vi "ReversedEngineering EvaluateStateActions.vi"(1 "SubViNames":string[](array[string]), 2 "StateDiagramSerachActions":T2, 5 "error in":errorcluster) -> (15 "StateActions":string[](array[string]), 19 "error out":errorcluster)   [LabVIEW 2016]
uses:
  <resource>/Framework/Providers/Open_GDS/UML/ReversedEngineering/ReversedEngineering StateAnalyseVIAction.ctl
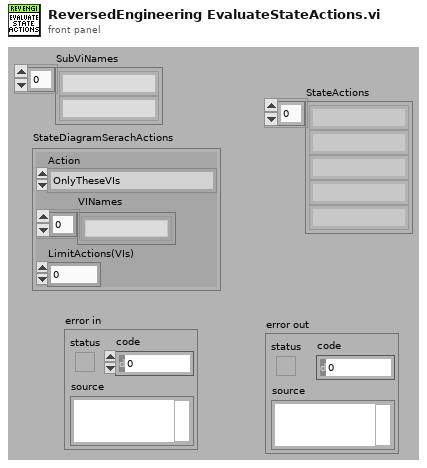
[diagram p1: front panel]
types:
  T1 = typedef "ReversedEngineering StateAnalyseVIAction.ctl" = enum16{"OnlyTheseVIs", "NotTheseVIs"}
  T2 = cluster{"Action":T1, "VINames":string[], "LimitActions(VIs)":i32}
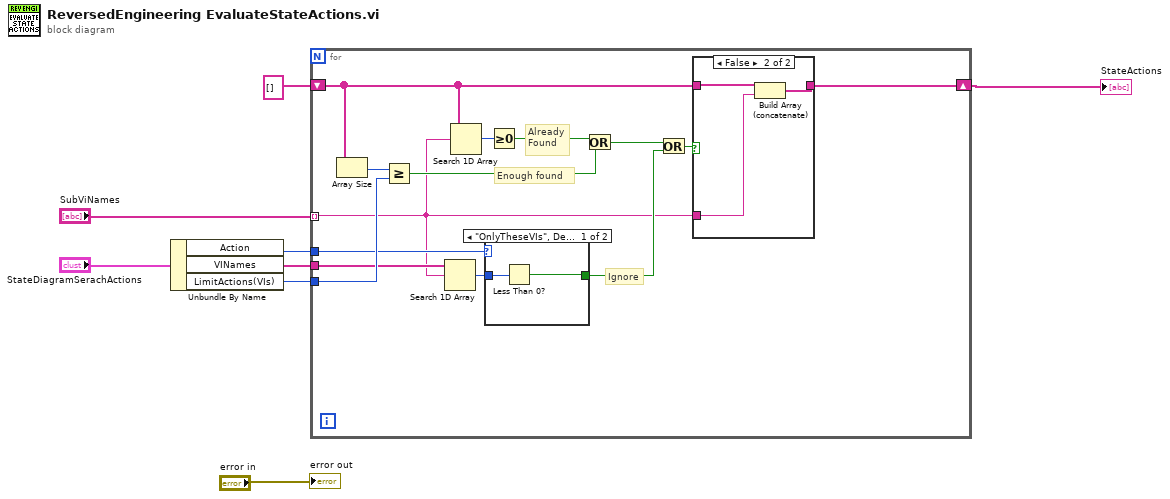
[diagram p0: block diagram]
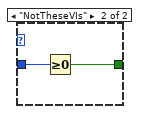
[diagram p2: hidden frame]
diagram:
  n1 = Unbundle By Name("StateDiagramSerachActions") -> ("Action"=w1:T1, "VINames"=w2:string[], "LimitActions(VIs)"=w3:i32)
  n2 = for {
    shift-right: [w22] -> w4
    shift-left: string[] [] ("StateActions") -> [w19]
    tunnel: "SubViNames" -> [w9] mode=indexing
    tunnel: w3 -> [w16]
    tunnel: w2 -> [w14]
    tunnel: w1 -> [w12]
    # "Ignore"
    # "Enough found"
    # "Already\nFound"
    n3 = Array Size(array=w19) -> (size(s)=w17:i32)
    n4 = Greater Or Equal?(x=w17, y=w16) -> (x >= y?=w15:bool)
    n5 = Search 1D Array(1D array=w14, element=w9) -> (index of element=w13:i32)  [unwired: 1 out]
    n6 = Search 1D Array(1D array=w19, element=w9) -> (index of element=w21:i32)  [unwired: 1 out]
    n7 = case shown="\"OnlyTheseVIs\", Default" w12 {
      tunnel: w13 -> [w24 w26]
      tunnel: [w23 w25] -> w10
      frame "OnlyTheseVIs", Default {
        n8 = Less Than 0?(x=w24) -> (x < 0?=w23:bool)
      }
      frame "NotTheseVIs" {
        n9 = Greater Or Equal To 0?(x=w26) -> (x >= 0?=w25:bool)
      }
    }
    n10 = Greater Or Equal To 0?(x=w21) -> (x >= 0?=w20:bool)
    n11 = Or(x=w20, y=w15) -> (x .or. y?=w18:bool)
    n12 = Or(x=w18, y=w10) -> (x .or. y?=w11:bool)
    n13 = case shown="False" w11 {
      tunnel: w19 -> [w27 w30]
      tunnel: [w27 w29] -> w22
      tunnel: w9 -> [_ w28]
      frame True {
        # "Ignored"
      }
      frame False {
        n14 = Build Array (concatenate)(w30, w28) -> (w29:string[])
      }
    }
  }
  "StateActions" <- w4
  "error out" <- "error in"
